vi "Close DC Loads.vi"(8 "Error in":errorcluster caption="Error in (no error)", 11 "DC Loads":refnum<class "Instrument.lvclass">[](array[class])) -> (0 "Error out":errorcluster)   [LabVIEW 2015, in "Instrument Close.lvclass"]
uses:
  Instrument Close.lvclass
  Classes/Instruments/Instrument/Class/Instrument.lvclass
  Classes/Instruments/DC Load/DC Load/Class/DC Load.lvclass
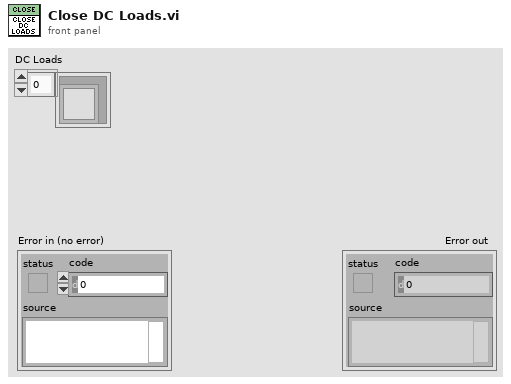
[diagram p1: front panel]
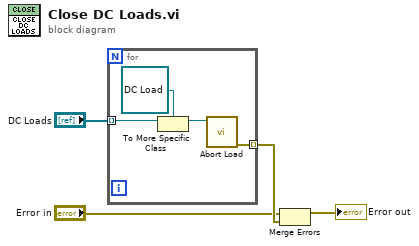
[diagram p0: block diagram]
diagram:
  n1 = for {
    tunnel: "DC Loads" -> [w8] mode=indexing
    tunnel: [w5] -> w3 mode=indexing
    n2 = To More Specific Class(target class=refnum<class "DC Load.lvclass"> refnum ("DC Load out"), reference=w8) -> (specific class reference=w6:refnum<class "DC Load.lvclass">)  [unwired: 1 in, 1 out]
    n3 = call-dynamic "Abort Load.vi"("DC Load in"=w6) -> ("error out"=w5:errorcluster)  [unwired: 9 in, 1 out]
  }
  n4 = Merge Errors("Error in", w3) -> (→"Error out":errorcluster)
